vi "NI DAQ stop.vi"(8 "error in":errorcluster, 11 "DAQmx Device Name":tag="PXI2Slot6") -> (0 "error out":errorcluster, 3 "DAQmx Device Name Out":tag="PXI2Slot6")   [LabVIEW 2020]
uses:
  <vilib>/DAQmx/write.llb/DAQmx Write (Analog 1D DBL 1Chan NSamp).vi
  NI DAQ globals.vi
  <vilib>/DAQmx/create/channels.llb/DAQmx Create Channel (AO-Voltage-Basic).vi
  <vilib>/DAQmx/configure/timing.llb/DAQmx Timing (Sample Clock).vi
  <vilib>/DAQmx/miscellaneous.llb/DAQmx Fill In Error Info.vi
  <resource>/objmgr/daqmx.rc
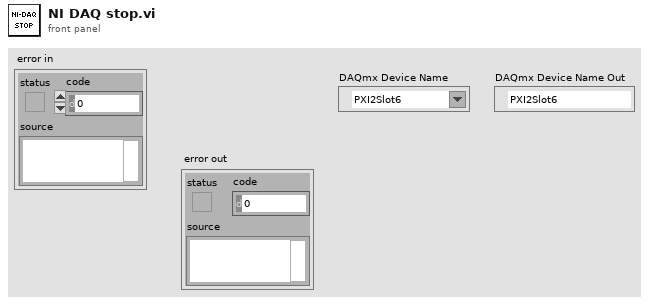
[diagram p1: front panel]
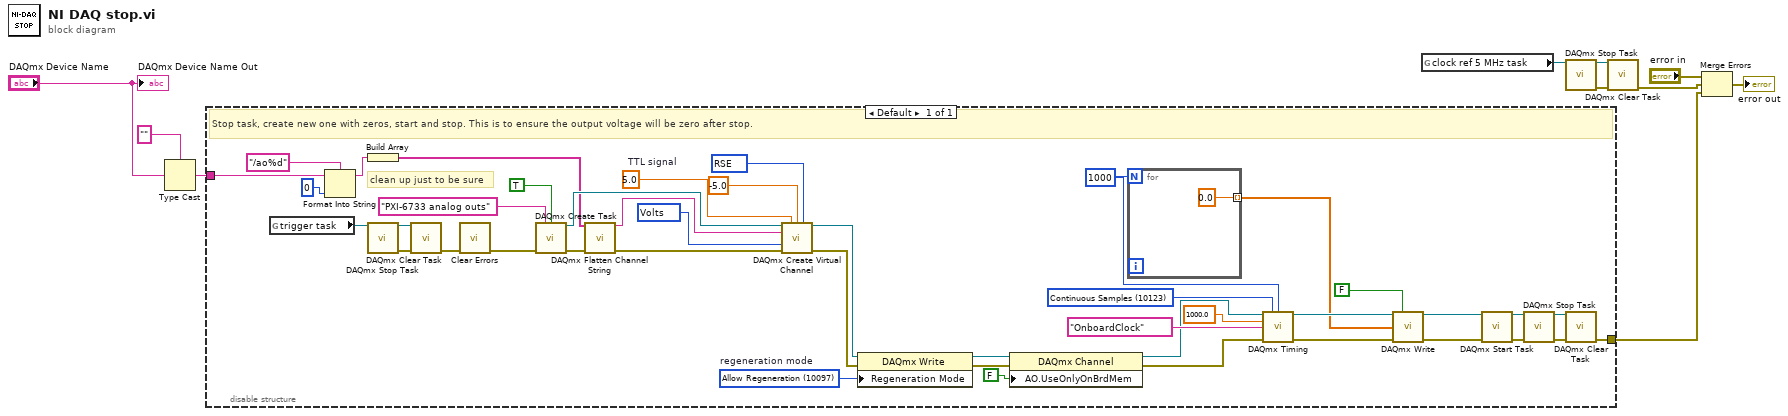
[diagram p0: block diagram]
diagram:
  n1 = Type Cast(type="", x="DAQmx Device Name") -> (*(type *) &x=w1:string)
  n2 = disable-structure shown="Default" {
    disable-tunnel: [w14] -> w4
    disable-tunnel: w1 -> [w13]
    frame Enabled {
      w11 = 1000 ("samples per channel")
      w26 = 10123 items=["Finite Samples"=10178, "Continuous Samples"=10123, "Hardware Timed Single Point"=12522] ("sample mode")
      w36 = 5.0  # TTL signal
      w46 = 10097 items=["Allow Regeneration"=10097, "Do Not Allow Regeneration"=10158]  # regeneration mode
      w47 = 10348 items=["Volts"=10348, "From Custom Scale"=10065] ("units")
      w48 = 10083 items=["Default"=-1, "RSE"=10083, "Differential"=10106, "Pseudodifferential"=12529] ("output terminal configuration")
      # "clean up just to be sure"
      # "Stop task, create new one with zeros, start and stop. This is to ensure the output voltage will be zero after stop."
      n3 = global read "NI DAQ globals.vi" "trigger task"() -> (w33:refnum<k21>)
      n4 = Format Into String(format string="/ao%d", initial string=w13, 0 ("input 1")) -> (resulting string=w38:string)  [unwired: 1 in, 1 out]
      n5 = Build Array(w38) -> (w37:string[])
      n6 = call <vilib>:"DAQmx Stop Task.vi"("task/channels in"=w33) -> ("task out"=w34:refnum<k21>, "error out"=w32:errorcluster)  [unwired: 13 in]
      n7 = call <vilib>:"DAQmx Clear Task.vi"("task in"=w34, "error in"=w32) -> ("error out"=w31:errorcluster)  [unwired: 13 in]
      n8 = call <vilib>:"Clear Errors.vi"("error in (no error)"=w31) -> ("error out"=w30:errorcluster)  [unwired: 5 in, 1 out]
      n9 = call <vilib>:"DAQmx Create Task.vi"("new task name"="PXI-6733 analog outs", "auto cleanup"=TRUE, "error in"=w30) -> ("task out"=w52:refnum<k21>, "error out"=w51:errorcluster)  [unwired: 11 in]
      n10 = call <vilib>:"DAQmx Flatten Channel String.vi"("names in"=w37, "error in"=w51) -> ("names out"=w49:string, "error out"=w50:errorcluster)  [unwired: 12 in]
      n11 = call-poly <vilib>:"DAQmx Create Virtual Channel.vi"("task in"=w52, "maximum value"=w36, "minimum value"=-5.0, "output terminal configuration"=w48, "physical channels"=w49, "units"=w47, "error in"=w50) -> ("task out"=w44:refnum<k21>, "error out"=w45:errorcluster)  [unwired: 7 in]
      n12 = property class="DAQmx Write"(reference=w44, error in=w45, "Regeneration Mode"=w46) -> (reference out=w41:refnum<k21>, error out=w42:errorcluster)
      n13 = property class="DAQmx Channel"(reference=w41, error in=w42, "AO.UseOnlyOnBrdMem"=FALSE) -> (reference out=w24:refnum<k21>, error out=w23:errorcluster)
      n14 = for {
        N: w11 -> [_]
        tunnel: [0.0 ("rate")] -> w12 mode=indexing
      }
      n15 = call-poly <vilib>:"DAQmx Timing.vi"("task/channels in"=w24, "sample mode"=w26, "samples per channel"=w11, "rate"=1000.0, "source"=tag "OnboardClock", "error in"=w23) -> ("task out"=w29:refnum<k21>, "error out"=w28:errorcluster)  [unwired: 8 in]
      n16 = call-poly <vilib>:"DAQmx Write.vi"("task/channels in"=w29, "auto start"=FALSE, "data"=w12, "error in"=w28) -> ("task out"=w16:refnum<k21>, "error out"=w18:errorcluster)  [unwired: 9 in, 1 out]
      n17 = call <vilib>:"DAQmx Start Task.vi"("task/channels in"=w16, "error in"=w18) -> ("task out"=w15:refnum<k21>, "error out"=w17:errorcluster)  [unwired: 12 in]
      n18 = call <vilib>:"DAQmx Stop Task.vi"("task/channels in"=w15, "error in"=w17) -> ("task out"=w19:refnum<k21>, "error out"=w20:errorcluster)  [unwired: 12 in]
      n19 = call <vilib>:"DAQmx Clear Task.vi"("task in"=w19, "error in"=w20) -> ("error out"=w14:errorcluster)  [unwired: 13 in]
    }
  }
  n20 = global read "NI DAQ globals.vi" "clock ref 5 MHz task"() -> (w6:refnum<k21>)
  n21 = call <vilib>:"DAQmx Stop Task.vi"("task/channels in"=w6) -> ("task out"=w7:refnum<k21>, "error out"=w8:errorcluster)  [unwired: 13 in]
  n22 = call <vilib>:"DAQmx Clear Task.vi"("task in"=w7, "error in"=w8) -> ("error out"=w5:errorcluster)  [unwired: 13 in]
  n23 = Merge Errors("error in", w5, w4) -> (→"error out":errorcluster)
  "DAQmx Device Name Out" <- "DAQmx Device Name"
